vi "Save Data.vi"(8 "error in (no error)":errorcluster, 10 "User Specified":T1={"Hardware Configuration"={"Signal Channel"="PXI1Slot7/ao0", "Response Channel"="PXI1Slot7/ai0", "Trigger Channel"="/PXI1Slot7/PFI0", "Number of Acquisitions"=0.0}, "Analysis Configuration"={"Statistics"=TRUE}, "Signal Type"=enum."Single Chirp", "New Data Behavior"=enum."Replace", "Signal Configuration"={"Chirp Amplitude"=0.1, "I/O Limit"=10.0, "Sample Rate"=1000000.0, "Chirp Duration (s)"=10000000.0, "Upper Frequency"=0.0, "Lower Frequency"=0.0, "Windowing"=enum."None"}, "Waveform File"="", "Save Location"=""}, 11 "Data":waveform(dbl)[](array[waveform])) -> (0 "error out":errorcluster)   [LabVIEW 2017]
doc: "Saves data to disk in the TDMS file format."
uses:
  controls/User Specified Data.ctl
  controls/HW Configuration.ctl
  controls/Analysis Configuration.ctl
  controls/New Data Behavior.ctl
  controls/Signal Configuration.ctl
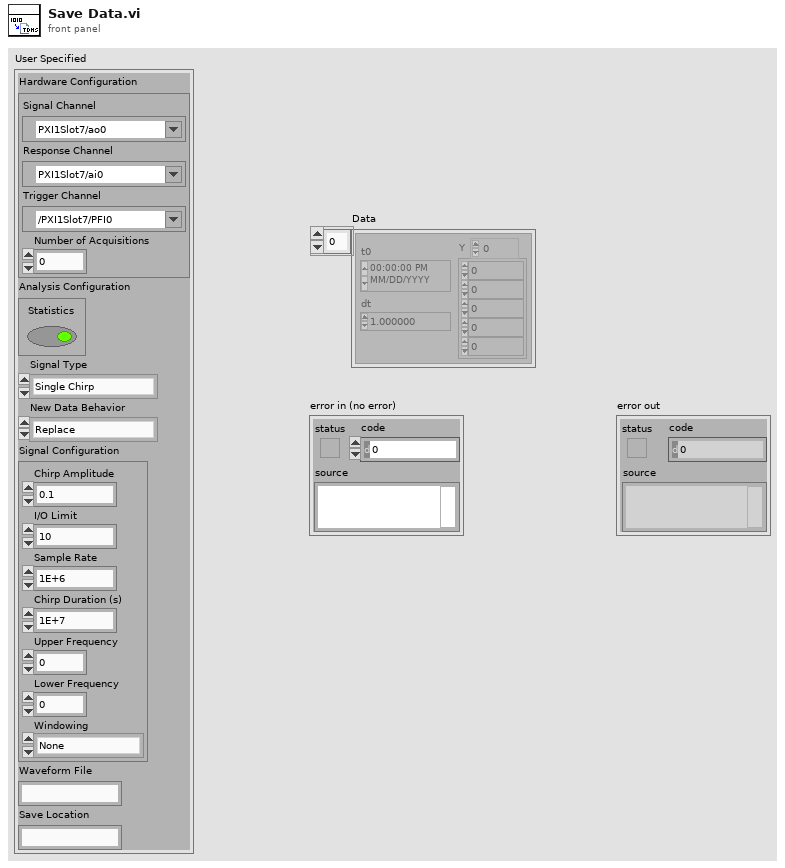
[diagram p1: front panel]
types:
  T1 = typedef "User Specified Data.ctl" = cluster{"Hardware Configuration":T2, "Analysis Configuration":T3, "Signal Type":enum16{"Single Chirp", "From Excel"}, "New Data Behavior":T4, "Signal Configuration":T5, "Waveform File":string, "Save Location":string}
  T2 = typedef "HW Configuration.ctl" = cluster{"Signal Channel":tag, "Response Channel":tag, "Trigger Channel":tag, "Number of Acquisitions":dbl}
  T3 = typedef "Analysis Configuration.ctl" = cluster{"Statistics":bool}
  T4 = typedef "New Data Behavior.ctl" = enum16{"Replace", "Overlay", "Append"}
  T5 = typedef "Signal Configuration.ctl" = cluster{"Chirp Amplitude":dbl, "I/O Limit":dbl, "Sample Rate":dbl, "Chirp Duration (s)":dbl, "Upper Frequency":dbl, "Lower Frequency":dbl, "Windowing":enum16{"None", "Exponential", "Flat top", "Hamming", "Hanning", "Kaiser-Bessel", "Rectangular"}}
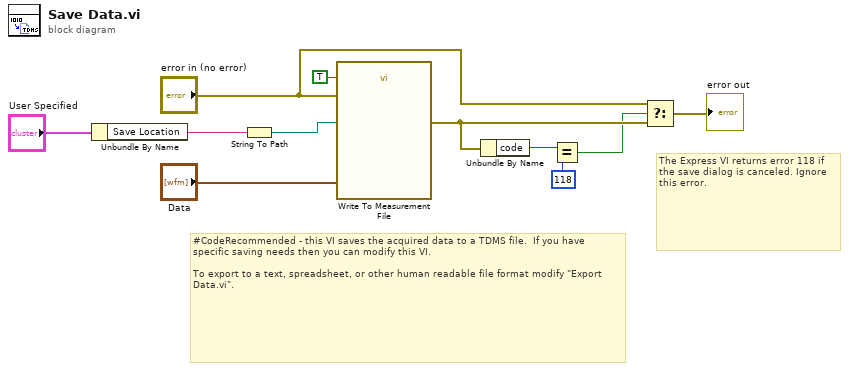
[diagram p0: block diagram]
diagram:
  # "The Express VI returns error 118 if the save dialog is canceled. Ignore this error."
  # "#CodeRecommended - this VI saves the acquired data to a TDMS file.  If you have specific saving needs then you can modify this VI.\n\nTo export to a text, spreadsheet, or other human readable file format modify \"Export Data.vi\"."
  n1 = Unbundle By Name("User Specified") -> ("Save Location"=w1:string)
  n2 = String To Path(string=w1) -> (path=w3:path)
  n3 = call "Write To Measurement File"("Signals"="Data", "Reset"=TRUE, "error in (no error)"="error in (no error)", "Filename"=w3) -> ("error out"=w8:errorcluster)  [unwired: 13 in, 2 out]
  n4 = Unbundle By Name(w8) -> ("code"=w6:i32)
  n5 = Equal?(x=w6, y=118) -> (x = y?=w5:bool)
  n6 = Select(t="error in (no error)", s=w5, f=w8) -> (s? t:f=→"error out":errorcluster)
